vi "Write Sorting Enabled.vi"(8 "error in":errorcluster, 10 "sort type":T1, 11 "EngineTags in":refnum<class "EngineTags.lvclass">) -> (0 "error out":errorcluster, 3 "EngineTags out":refnum<class "EngineTags.lvclass">)   [LabVIEW 2013, in "PL Framework Configuration Tool.lvlib" / "EngineTags.lvclass"]
uses:
  EngineTags.lvclass
  sorting type.ctl
  EngineTags.lvclass/EngineTags.ctl
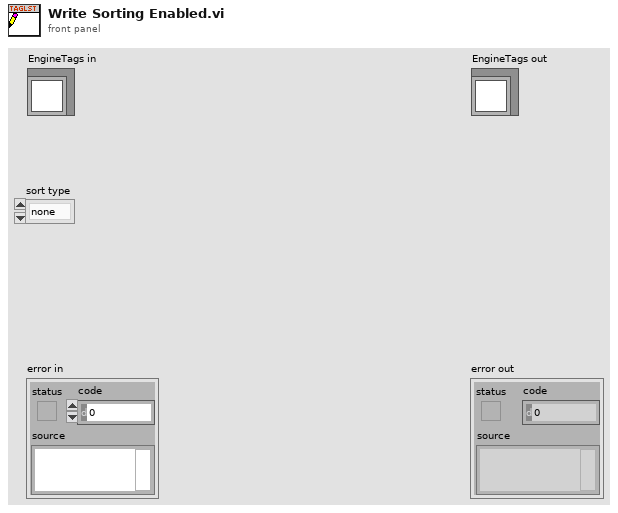
[diagram p1: front panel]
types:
  T1 = typedef "PL Framework Configuration Tool.lvlib/EngineTags.lvclass/sorting type.ctl" = enum16{"none", "asc", "desc"}
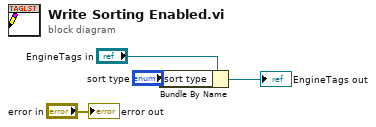
[diagram p0: block diagram]
diagram:
  n1 = Bundle By Name(cluster="EngineTags in", "sort type"="sort type") -> (→"EngineTags out":refnum<class "EngineTags.lvclass">)
  "error out" <- "error in"
